vi "Actor Core.vi"(8 "error in":errorcluster, 11 "Main_UI in":refnum<class "Main_UI.lvclass">) -> (0 "error out":errorcluster, 3 "Actor out":refnum<class "Actor.lvclass">)   [LabVIEW 2020, in "Main_UI.lvlib" / "Main_UI.lvclass"]
doc: "(<B>Filename</B>: Actor Framework.lvlib:Actor.lvclass:Actor Core.vi)\n\nReceives messages to the actor, reacts to them, and initiates any error handling that may shut the actor down.\n\nDescendant classes may override this VI to append parallel tasks for the actor to complete while it handles messages. Overrides use the Call Parent Class Method node."
uses:
  Main_UI.lvclass
  C:/Program Files/National Instruments/LabVIEW 2020/vi.lib/ActorFramework/Actor/Actor.lvclass
  <vilib>/ActorFramework/Actor/Actor.lvclass
  <vilib>/ActorFramework/Actor/Actor.lvclass/Actor.ctl
  <vilib>/ActorFramework/Message Enqueuer/Message Enqueuer.lvclass/Message Enqueuer.ctl
  Main_UI.lvclass/Main_UI.ctl
  <vilib>/ActorFramework/Stop Msg/Stop Msg.lvclass/Stop Msg.ctl
  <vilib>/ActorFramework/Message Enqueuer/Init from Existing Queue.vi
  <vilib>/ActorFramework/Stop Msg/Send Emergency Stop.vi
  <vilib>/ActorFramework/Stop Msg/Send Normal Stop.vi
  <vilib>/ActorFramework/Message Enqueuer/Enqueue.vi
  <vilib>/ActorFramework/Message Enqueuer/Enqueue Critical.vi
  <vilib>/ActorFramework/Stop Msg/Stop Msg.lvclass
  C:/Program Files/National Instruments/LabVIEW 2020/vi.lib/ActorFramework/Message/Message.lvclass
  IUI_Command Messages/cmd Stop Msg/cmd Stop Msg.lvclass
  IUI_Command Messages/cmd RandGen Msg/cmd RandGen Msg.lvclass
  <vilib>/ActorFramework/Message Priority Queue/Priority Enqueue.vi
  <vilib>/ActorFramework/Message Enqueuer/Message Enqueuer.lvclass
panel:
  in  "Btn Exit":bool
  in  "Btn Rand Gen":bool
  out "Random Number Display":dbl
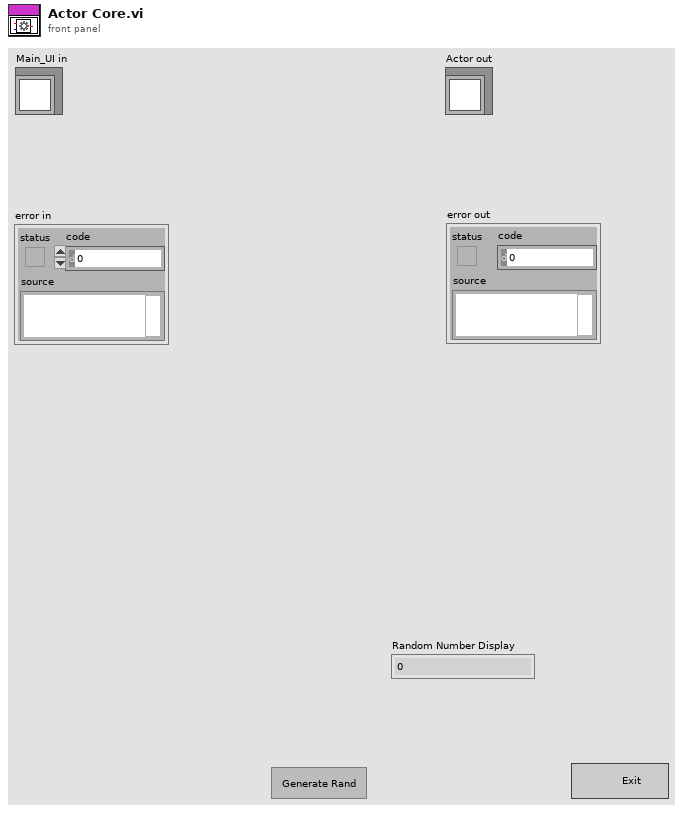
[diagram p1: front panel]
types:
  T1 = enum32{"Invalid", "Standard", "Closed", "Hidden", "Minimized", "Maximized"}
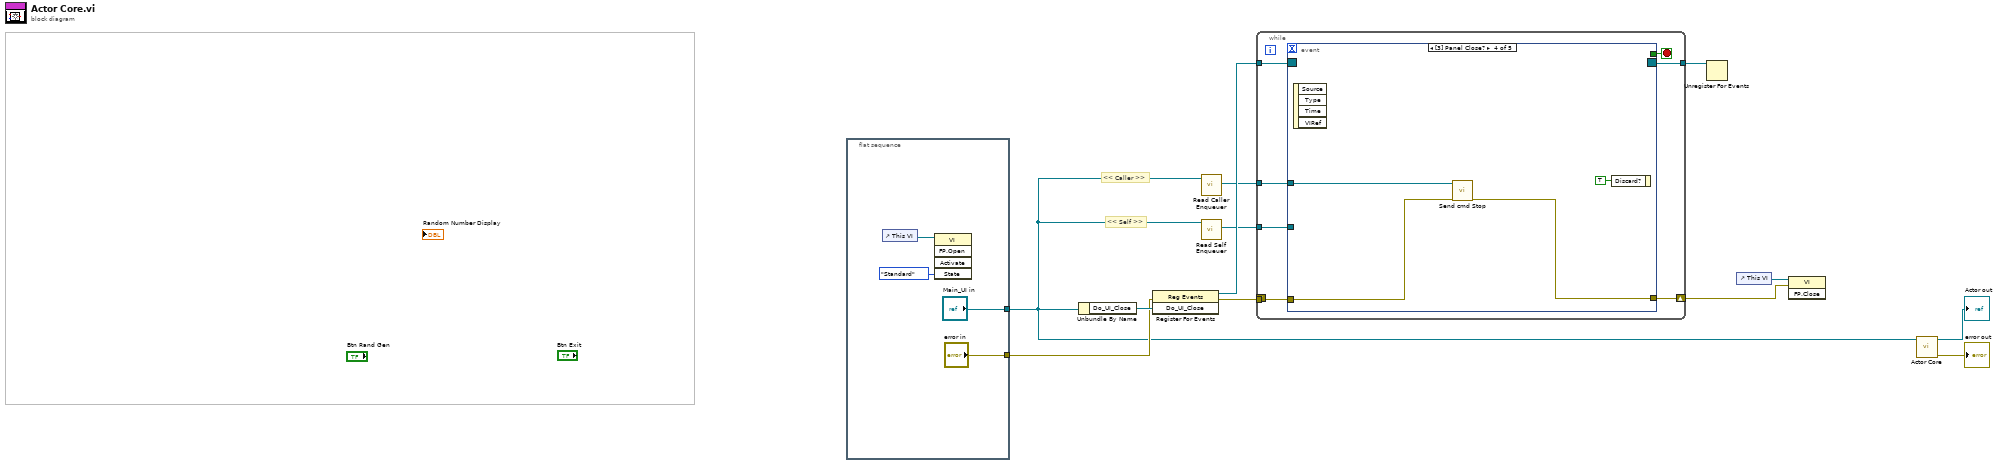
[diagram p0: block diagram]
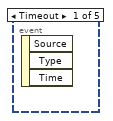
[diagram p2: hidden frame]
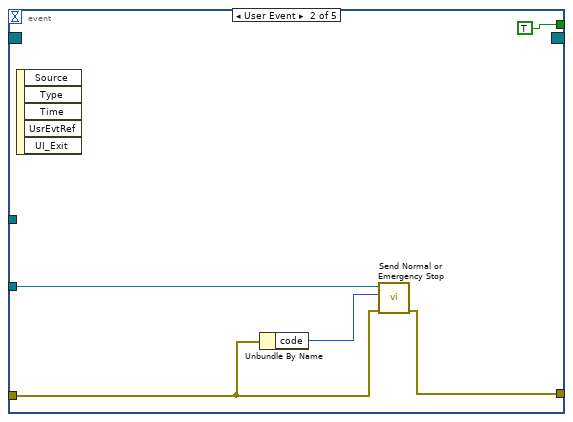
[diagram p3: hidden frame]
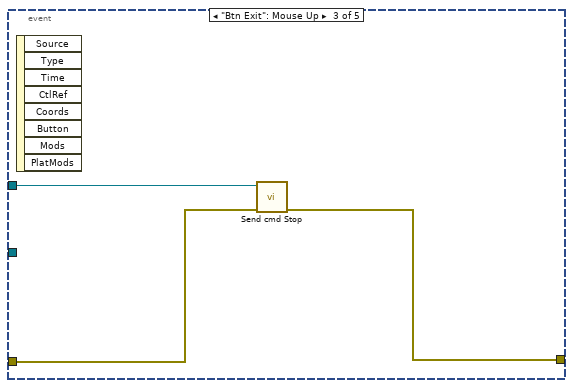
[diagram p4: hidden frame]
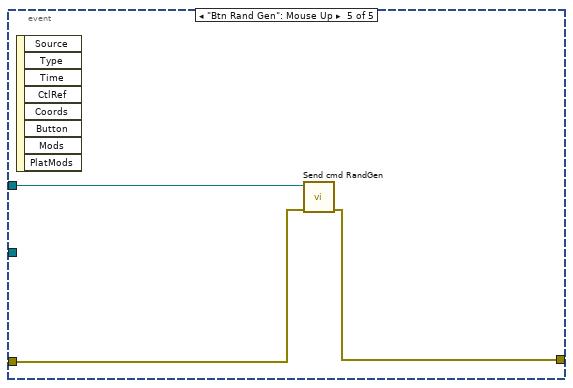
[diagram p5: hidden frame]
diagram:
  # "<< Self >>"
  # "<< Caller >>"
  n1 = flat-sequence {
    tunnel: ["error in"] -> w7
    tunnel: ["Main_UI in"] -> w3
    frame #0 {
      n2 = control-ref of="This VI"() -> (w14:refnum<vi>)
      n3 = invoke class="VI" method="FP.Open"(reference=w14, "State"=T1."Standard") -> ()  [unwired: 3 in, 5 out]
    }
  }
  n4 = Unbundle By Name(w3) -> ("Do_UI_Close"=w10:refnum<user-event>)
  n5 = register-events(error in=w7, w10) -> (reference out=w9:refnum<event-registration>, error out=w6:errorcluster)  [unwired: 1 in]
  n6 = call <vilib>:"Read Caller Enqueuer.vi"("Actor"=w3) -> ("Caller Enqueuer"=w5:refnum<class "Message Enqueuer.lvclass">)  [unwired: 10 in]
  n7 = call <vilib>:"Read Self Enqueuer.vi"("Actor"=w3) -> ("Self Enqueuer"=w4:refnum<class "Message Enqueuer.lvclass">)  [unwired: 10 in]
  n8 = while {
    tunnel: w9 -> [w23]
    tunnel: [w21] -> w8
    tunnel: w6 -> [w20]
    tunnel: w5 -> [w19]
    tunnel: w4 -> [w18]
    shift-right: [w17] -> w1
    shift-left: _ -> [_]
    stop <- w22 stop-if-true
    n9 = event shown="[3] Panel Close?" {
      selector: w23 -> [_ _ _ _ _]
      dyn-events: [_ _ _ _ _] -> w21
      timeout: _ -> [_ _ _ _ _]
      tunnel: [_ TRUE _ _ _] -> w22
      tunnel: w20 -> [_ w26 w30 w34 w37]
      tunnel: w19 -> [_ _ w31 w35 w38]
      tunnel: w18 -> [_ w24 _ _ _]
      tunnel: [_ w25 w29 w33 w36] -> w17
      event Timeout {
        n10 = event-data() -> ()  [unwired: 1 in, 3 out]
      }
      event User Event {
        n11 = event-data() -> ()  [unwired: 1 in, 5 out]
        n12 = Unbundle By Name(w26) -> ("code"=w27:i32)
        n13 = call <vilib>:"Send Normal or Emergency Stop.vi"("error in (no error)"=w26, "final error code"=w27, "Message Enqueuer"=w24) -> ("error out"=w25:errorcluster)  [unwired: 8 in]
      }
      event "Btn Exit": Mouse Up {
        n14 = event-data() -> ()  [unwired: 1 in, 8 out]
        n15 = call "Send cmd Stop.vi"("error in (no error)"=w30, "Message Enqueuer"=w31) -> ("error out"=w29:errorcluster)  [unwired: 8 in, 1 out]
      }
      event Panel Close? {
        n16 = event-data() -> ()  [unwired: 1 in, 4 out]
        n17 = call "Send cmd Stop.vi"("error in (no error)"=w34, "Message Enqueuer"=w35) -> ("error out"=w33:errorcluster)  [unwired: 8 in, 1 out]
        n18 = event-data("Discard?"=TRUE) -> ()  [unwired: 1 in, 1 out]
      }
      event "Btn Rand Gen": Mouse Up {
        n19 = event-data() -> ()  [unwired: 1 in, 8 out]
        n20 = call "Send cmd RandGen.vi"("error in (no error)"=w37, "Message Enqueuer"=w38) -> ("error out"=w36:errorcluster)  [unwired: 8 in, 1 out]
      }
    }
  }
  n21 = Unregister For Events(event registration refnum=w8) -> ()  [unwired: 1 in, 1 out]
  n22 = control-ref of="This VI"() -> (w2:refnum<vi>)
  n23 = invoke class="VI" method="FP.Close"(reference=w2, error in=w1) -> ()  [unwired: 1 in, 3 out]
  n24 = call-parent "Actor Core.vi"("Actor in"=w3) -> ("error out"=→"error out":errorcluster, "Actor out"=→"Actor out":refnum<class "Actor.lvclass">)  [unwired: 9 in]
